vi "RANGE Configuration File.vi"(7 "Debug":bool, 8 "Error In":errorcluster, 11 "Gas Lab Config File":path=path "C:/Technology Lab/NI-2010/Trunk/Range/Documentation/GasLabConfigurationFile.txt") -> (0 "Error Out":errorcluster, 3 "Meter Data":T2={"Meter 1"={"Meter Size"=0.0, "DAQ Output (Voltage)"=0.0, "Reference (Voltage)"=0.0, "Meter Present"=FALSE, "Meter Visa"="COM3", "Gas Type"="", "SLPM Error @ Zero"=0.0, "Gas Mix Number"="", "Set STP Register"=FALSE, "Measurement Units"={"Abs. Pressure"="", "Gauge/Diff. Press."="", "Barometric Press."="", "Temperature"="", "Volume"="", "Mass"="", "Setpoint"="", "Valve Drive"="", "Totalizer"="", "Tot. Timer"="", "Tot. Avg. Flow"="", "Tot. Peak Flow"="", "Software Version"=""}}, "Meter 2"={"Meter Size"=0.0, "DAQ Output (Voltage)"=0.0, "Reference (Voltage)"=0.0, "Meter Present"=FALSE, "Meter Visa"="COM3", "Gas Type"="", "SLPM Error @ Zero"=0.0, "Gas Mix Number"="", "Set STP Register"=FALSE, "Measurement Units"={"Abs. Pressure"="", "Gauge/Diff. Press."="", "Barometric Press."="", "Temperature"="", "Volume"="", "Mass"="", "Setpoint"="", "Valve Drive"="", "Totalizer"="", "Tot. Timer"="", "Tot. Avg. Flow"="", "Tot. Peak Flow"="", "Software Version"=""}}, "Meter 3"={"Meter Size"=0.0, "DAQ Output (Voltage)"=0.0, "Reference (Voltage)"=0.0, "Meter Present"=FALSE, "Meter Visa"="COM3", "Gas Type"="", "SLPM Error @ Zero"=0.0, "Gas Mix Number"="", "Set STP Register"=FALSE, "Measurement Units"={"Abs. Pressure"="", "Gauge/Diff. Press."="", "Barometric Press."="", "Temperature"="", "Volume"="", "Mass"="", "Setpoint"="", "Valve Drive"="", "Totalizer"="", "Tot. Timer"="", "Tot. Avg. Flow"="", "Tot. Peak Flow"="", "Software Version"=""}}, "Meter 4"={"Meter Size"=0.0, "DAQ Output (Voltage)"=0.0, "Reference (Voltage)"=0.0, "Meter Present"=FALSE, "Meter Visa"="COM3", "Gas Type"="", "SLPM Error @ Zero"=0.0, "Gas Mix Number"="", "Set STP Register"=FALSE, "Measurement Units"={"Abs. Pressure"="", "Gauge/Diff. Press."="", "Barometric Press."="", "Temperature"="", "Volume"="", "Mass"="", "Setpoint"="", "Valve Drive"="", "Totalizer"="", "Tot. Timer"="", "Tot. Avg. Flow"="", "Tot. Peak Flow"="", "Software Version"=""}}, "Meter 5"={"Meter Size"=0.0, "DAQ Output (Voltage)"=0.0, "Reference (Voltage)"=0.0, "Meter Present"=FALSE, "Meter Visa"="COM3", "Gas Type"="", "SLPM Error @ Zero"=0.0, "Gas Mix Number"="", "Set STP Register"=FALSE, "Measurement Units"={"Abs. Pressure"="", "Gauge/Diff. Press."="", "Barometric Press."="", "Temperature"="", "Volume"="", "Mass"="", "Setpoint"="", "Valve Drive"="", "Totalizer"="", "Tot. Timer"="", "Tot. Avg. Flow"="", "Tot. Peak Flow"="", "Software Version"=""}}, "Meter 6"={"Meter Size"=0.0, "DAQ Output (Voltage)"=0.0, "Reference (Voltage)"=0.0, "Meter Present"=FALSE, "Meter Visa"="COM3", "Gas Type"="", "SLPM Error @ Zero"=0.0, "Gas Mix Number"="", "Set STP Register"=FALSE, "Measurement Units"={"Abs. Pressure"="", "Gauge/Diff. Press."="", "Barometric Press."="", "Temperature"="", "Volume"="", "Mass"="", "Setpoint"="", "Valve Drive"="", "Totalizer"="", "Tot. Timer"="", "Tot. Avg. Flow"="", "Tot. Peak Flow"="", "Software Version"=""}}, "Meter Bank 1"={"Flow Rate (BTU/HR)"=0.0, "ANSI Placeholder Array"=[], "15 Sec Avg Array"=[], "30 Sec Avg Array "=[], "ANSI Average (BTU/HR)"=0.0, "Panel Data"={"Meter Type (Gas)"="", "Heating Value (BTU/ft³)"=0.0, "Ft³ / Hr (SCFH)"=0.0, "15 Second Average (BTU/HR)"=0.0, "30 Second Average (BTU/HR)"=0.0, "Mass Flow"=0.0, "Vol. Flow"=0.0, "Gas Temperature"=0.0, "Gas Pressure"=0.0, "Tot.Flow"=0.0}, "Start ANSI"=FALSE, "ANSI Start Time"=0.0, "Restart ANSI"=FALSE, "Meter ID"=""}, "Meter Bank 2"={"Flow Rate (BTU/HR)"=0.0, "ANSI Placeholder Array"=[], "15 Sec Avg Array"=[], "30 Sec Avg Array "=[], "ANSI Average (BTU/HR)"=0.0, "Panel Data"={"Meter Type (Gas)"="", "Heating Value (BTU/ft³)"=0.0, "Ft³ / Hr (SCFH)"=0.0, "15 Second Average (BTU/HR)"=0.0, "30 Second Average (BTU/HR)"=0.0, "Mass Flow"=0.0, "Vol. Flow"=0.0, "Gas Temperature"=0.0, "Gas Pressure"=0.0, "Tot.Flow"=0.0}, "Start ANSI"=FALSE, "ANSI Start Time"=0.0, "Restart ANSI"=FALSE, "Meter ID"=""}, "Meter Bank 3"={"Flow Rate (BTU/HR)"=0.0, "ANSI Placeholder Array"=[], "15 Sec Avg Array"=[], "30 Sec Avg Array "=[], "ANSI Average (BTU/HR)"=0.0, "Panel Data"={"Meter Type (Gas)"="", "Heating Value (BTU/ft³)"=0.0, "Ft³ / Hr (SCFH)"=0.0, "15 Second Average (BTU/HR)"=0.0, "30 Second Average (BTU/HR)"=0.0, "Mass Flow"=0.0, "Vol. Flow"=0.0, "Gas Temperature"=0.0, "Gas Pressure"=0.0, "Tot.Flow"=0.0}, "Start ANSI"=FALSE, "ANSI Start Time"=0.0, "Restart ANSI"=FALSE, "Meter ID"=""}, "Threshold Voltage (NI DAQ)"=0.2, "Use RS232 Data Collection"=FALSE, "Use Auto Switching"=FALSE})   [LabVIEW 2018]
uses:
  Type Definitions/RANGE DAQ Data Four Meters.ctl
  Type Definitions/RANGE DAQ Data.ctl
  Drivers/Omega FMA-1600A Series Gas Flow Meter/Type Definitions/FMA1600A Gas Type.ctl
  Drivers/Omega FMA-1600A Series Gas Flow Meter/Type Definitions/FMA1600A Units String.ctl
  Type Definitions/RANGE GAS Data.ctl
  Type Definitions/RANGE Panel Data.ctl
panel:
  out "Meter 1.Measurement Units":T1
  out "all rows":string[][](array[string])
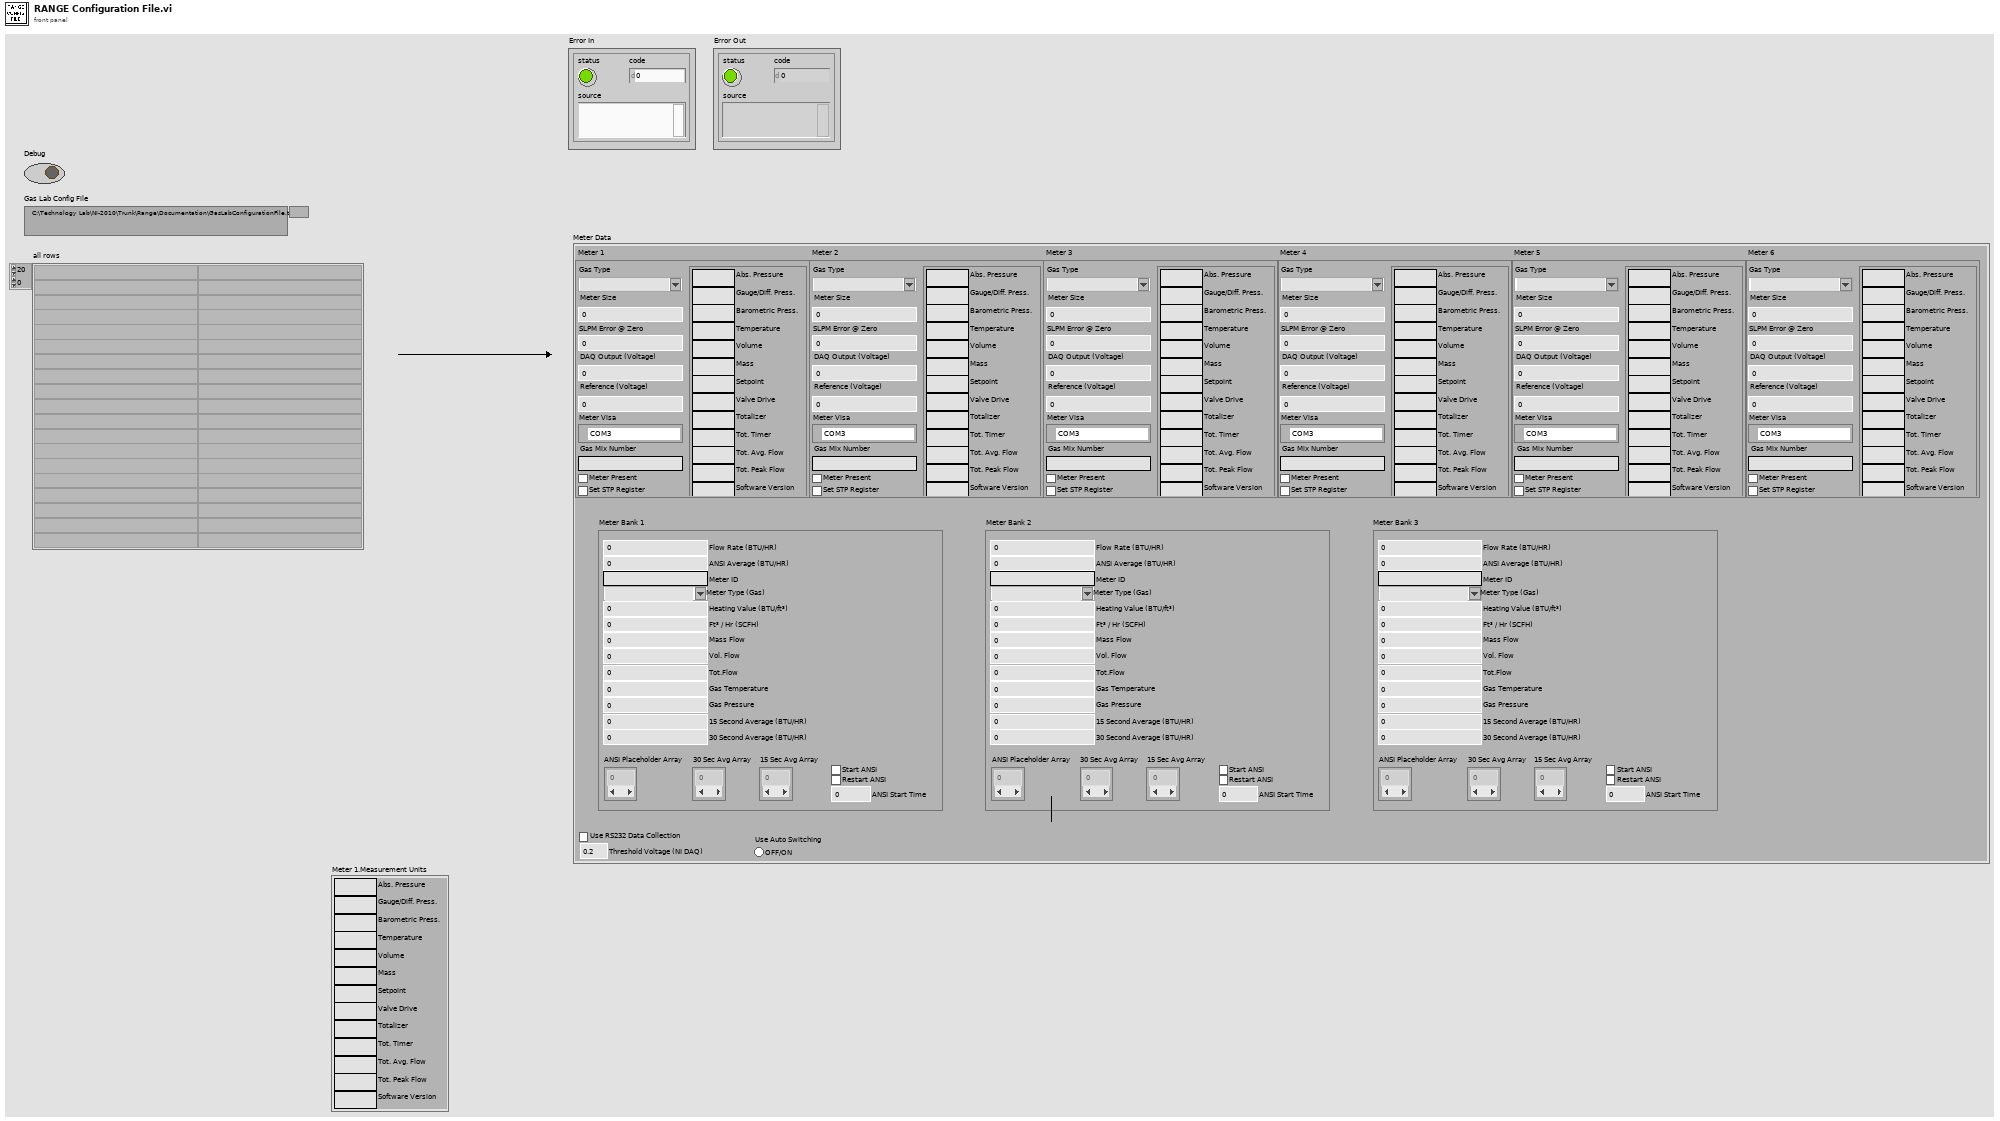
[diagram p1: front panel]
types:
  T1 = typedef "FMA1600A Units String.ctl" = cluster{"Abs. Pressure":string, "Gauge/Diff. Press.":string, "Barometric Press.":string, "Temperature":string, "Volume":string, "Mass":string, "Setpoint":string, "Valve Drive":string, "Totalizer":string, "Tot. Timer":string, "Tot. Avg. Flow":string, "Tot. Peak Flow":string, "Software Version":string}
  T2 = typedef "RANGE DAQ Data Four Meters.ctl" = cluster{"Meter 1":T3, "Meter 2":T3, "Meter 3":T3, "Meter 4":T3, "Meter 5":T3, "Meter 6":T3, "Meter Bank 1":T5, "Meter Bank 2":T5, "Meter Bank 3":T5, "Threshold Voltage (NI DAQ)":dbl, "Use RS232 Data Collection":bool, "Use Auto Switching":bool}
  T3 = typedef "RANGE DAQ Data.ctl" = cluster{"Meter Size":dbl, "DAQ Output (Voltage)":dbl, "Reference (Voltage)":dbl, "Meter Present":bool, "Meter Visa":refnum<visa-resource-name>, "Gas Type":T4, "SLPM Error @ Zero":dbl, "Gas Mix Number":string, "Set STP Register":bool, "Measurement Units":T1}
  T4 = typedef "FMA1600A Gas Type.ctl" = string
  T5 = typedef "RANGE GAS Data.ctl" = cluster{"Flow Rate (BTU/HR)":dbl, "ANSI Placeholder Array":dbl[], "15 Sec Avg Array":dbl[], "30 Sec Avg Array ":dbl[], "ANSI Average (BTU/HR)":dbl, "Panel Data":T6, "Start ANSI":bool, "ANSI Start Time":dbl, "Restart ANSI":bool, "Meter ID":string}
  T6 = typedef "RANGE Panel Data.ctl" = cluster{"Meter Type (Gas)":T4, "Heating Value (BTU/ft³)":dbl, "Ft³ / Hr (SCFH)":dbl, "15 Second Average (BTU/HR)":dbl, "30 Second Average (BTU/HR)":dbl, "Mass Flow":dbl, "Vol. Flow":dbl, "Gas Temperature":dbl, "Gas Pressure":dbl, "Tot.Flow":dbl}
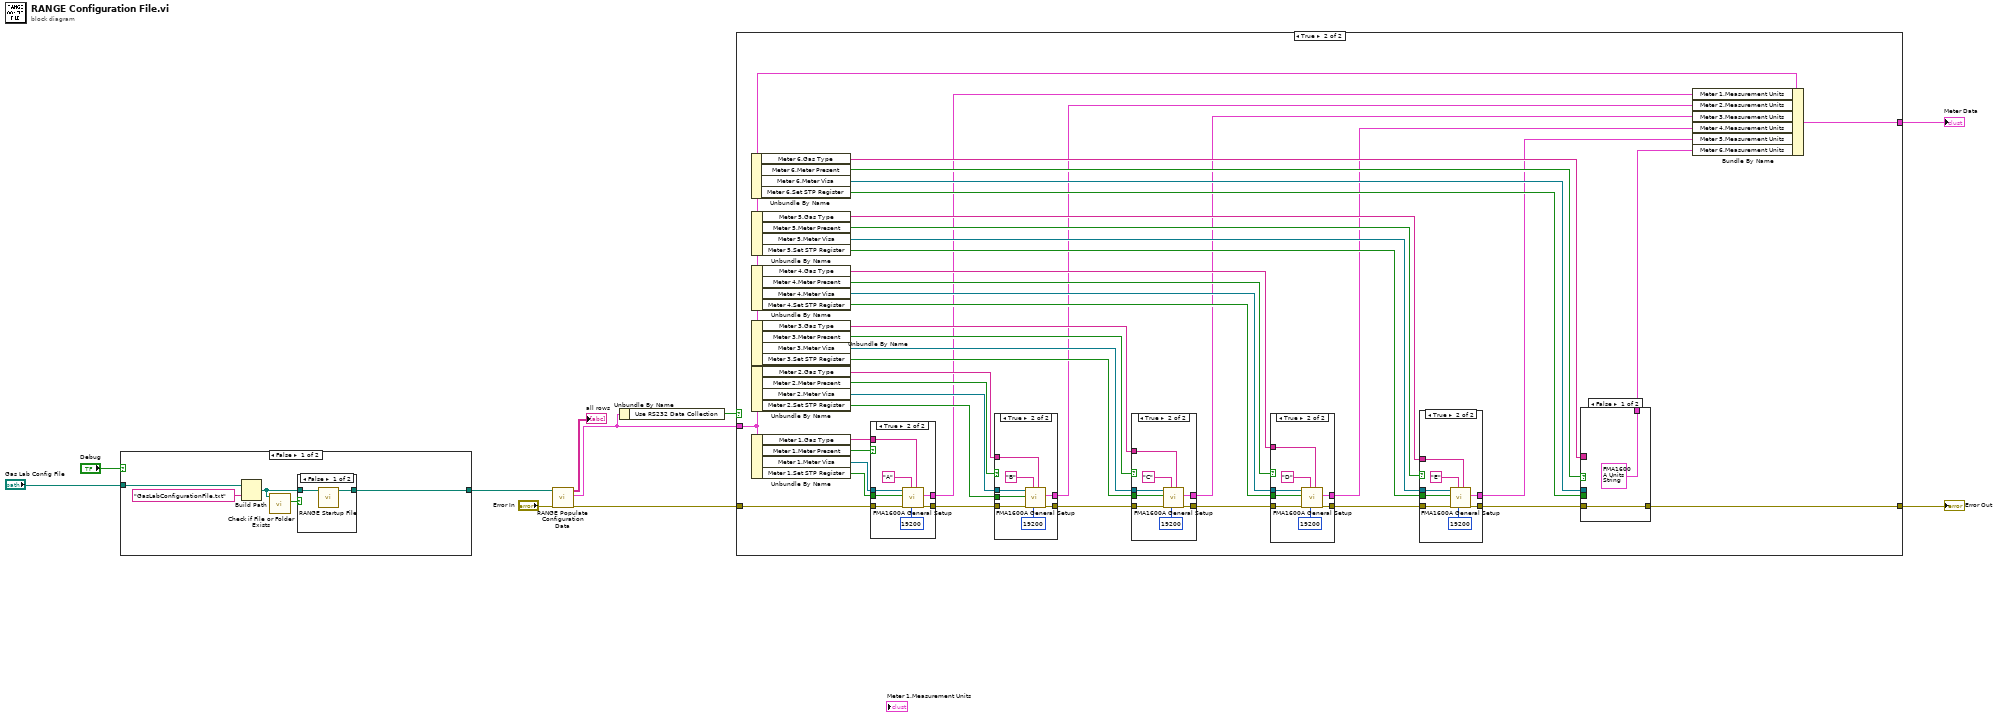
[diagram p0: block diagram]
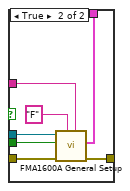
[diagram p3: hidden frame]
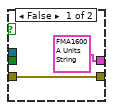
[diagram p4: hidden frame]
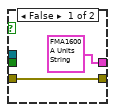
[diagram p5: hidden frame]
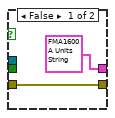
[diagram p6: hidden frame]
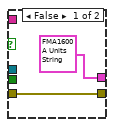
[diagram p7: hidden frame]
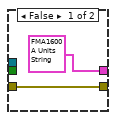
[diagram p8: hidden frame]
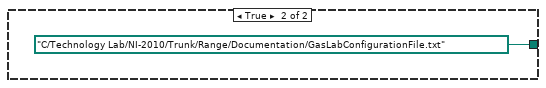
[diagram p10: hidden frame]
diagram:
  n1 = case shown="False" "Debug" {
    tunnel: "Gas Lab Config File" -> [w15 _]
    tunnel: [w11 path "C:/Technology Lab/NI-2010/Trunk/Range/Documentation/GasLabConfigurationFile.txt" ("appended path")] -> w8
    frame False {
      n2 = Build Path(base path=w15, name or relative path="GasLabConfigurationFile.txt") -> (appended path=w12:path)
      n3 = call <vilib>:"Check if File or Folder Exists.vi"("path"=w12) -> ("file or folder exists?"=w13:bool)  [unwired: 8 in, 2 out]
      n4 = case shown="False" w13 {
        tunnel: w12 -> [w17 w18]
        tunnel: [w16 w18] -> w11
        frame False {
          n5 = call "RANGE Startup File.vi"("appended path"=w17) -> ("new file path (Not A Path if cancelled)"=w16:path)  [unwired: 10 in]
        }
        frame True {
        }
      }
    }
    frame True {
    }
  }
  n6 = call "RANGE Populate Configuration Data.vi"("error in (no error)"="Error In", "appended path"=w8) -> ("error out"=w5:errorcluster, "DAQ Data"=w3:T2, "all rows"=→"all rows":string[][])  [unwired: 7 in]
  n7 = Unbundle By Name(w3) -> ("Use RS232 Data Collection"=w4:bool)
  n8 = case shown="True" w4 {
    tunnel: w5 -> [w21 w60]
    tunnel: w3 -> [w20 w29]
    tunnel: [w21 w52] -> w2
    tunnel: [w20 w22] -> w1
    frame False {
    }
    frame True {
      n9 = Unbundle By Name(w29) -> ("Meter 6.Gas Type"=w36:T4, "Meter 6.Meter Present"=w43:bool, "Meter 6.Meter Visa"=w42:refnum<visa-resource-name>, "Meter 6.Set STP Register"=w30:bool)
      n10 = Unbundle By Name(w29) -> ("Meter 5.Gas Type"=w37:T4, "Meter 5.Meter Present"=w45:bool, "Meter 5.Meter Visa"=w44:refnum<visa-resource-name>, "Meter 5.Set STP Register"=w31:bool)
      n11 = Unbundle By Name(w29) -> ("Meter 4.Gas Type"=w38:T4, "Meter 4.Meter Present"=w47:bool, "Meter 4.Meter Visa"=w46:refnum<visa-resource-name>, "Meter 4.Set STP Register"=w32:bool)
      n12 = Unbundle By Name(w29) -> ("Meter 3.Gas Type"=w39:T4, "Meter 3.Meter Present"=w49:bool, "Meter 3.Meter Visa"=w48:refnum<visa-resource-name>, "Meter 3.Set STP Register"=w33:bool)
      n13 = Unbundle By Name(w29) -> ("Meter 2.Gas Type"=w40:T4, "Meter 2.Meter Present"=w51:bool, "Meter 2.Meter Visa"=w50:refnum<visa-resource-name>, "Meter 2.Set STP Register"=w34:bool)
      n14 = Unbundle By Name(w29) -> ("Meter 1.Gas Type"=w41:T4, "Meter 1.Meter Present"=w59:bool, "Meter 1.Meter Visa"=w58:refnum<visa-resource-name>, "Meter 1.Set STP Register"=w35:bool)
      n15 = case shown="True" w59 {
        tunnel: w60 -> [w111 w119]
        tunnel: w58 -> [_ w118]
        tunnel: [w111 w116] -> w57
        tunnel: w41 -> [_ w115]
        tunnel: w35 -> [_ w114]
        tunnel: [T1 {"Abs. Pressure"="", "Gauge/Diff. Press."="", "Barometric Press."="", "Temperature"="", "Volume"="", "Mass"="", "Setpoint"="", "Valve Drive"="", "Totalizer"="", "Tot. Timer"="", "Tot. Avg. Flow"="", "Tot. Peak Flow"="", "Software Version"=""} ("Measurement Units") w113] -> w28
        frame False {
        }
        frame True {
          n16 = call "FMA1600A General Setup.vi"("Gas Type"=w115, "baud rate (19200)"=u32 19200, "Unit ID"="A", "error in (no error)"=w119, "Set STP Register"=w114, "VISA Refnum in"=w118) -> ("error out"=w116:errorcluster, "Measurement Units"=w113:T1)  [unwired: 3 in, 1 out]
        }
      }
      n17 = case shown="True" w51 {
        tunnel: w57 -> [w101 w109]
        tunnel: w50 -> [_ w108]
        tunnel: [w101 w106] -> w56
        tunnel: w40 -> [_ w105]
        tunnel: w34 -> [_ w104]
        tunnel: [T1 {"Abs. Pressure"="", "Gauge/Diff. Press."="", "Barometric Press."="", "Temperature"="", "Volume"="", "Mass"="", "Setpoint"="", "Valve Drive"="", "Totalizer"="", "Tot. Timer"="", "Tot. Avg. Flow"="", "Tot. Peak Flow"="", "Software Version"=""} ("Measurement Units") w103] -> w27
        frame False {
        }
        frame True {
          n18 = call "FMA1600A General Setup.vi"("Gas Type"=w105, "baud rate (19200)"=u32 19200, "Unit ID"="B", "error in (no error)"=w109, "Set STP Register"=w104, "VISA Refnum in"=w108) -> ("error out"=w106:errorcluster, "Measurement Units"=w103:T1)  [unwired: 3 in, 1 out]
        }
      }
      n19 = case shown="True" w49 {
        tunnel: w56 -> [w91 w99]
        tunnel: w48 -> [_ w98]
        tunnel: [w91 w96] -> w55
        tunnel: w39 -> [_ w95]
        tunnel: w33 -> [_ w94]
        tunnel: [T1 {"Abs. Pressure"="", "Gauge/Diff. Press."="", "Barometric Press."="", "Temperature"="", "Volume"="", "Mass"="", "Setpoint"="", "Valve Drive"="", "Totalizer"="", "Tot. Timer"="", "Tot. Avg. Flow"="", "Tot. Peak Flow"="", "Software Version"=""} ("Measurement Units") w93] -> w26
        frame False {
        }
        frame True {
          n20 = call "FMA1600A General Setup.vi"("Gas Type"=w95, "baud rate (19200)"=u32 19200, "Unit ID"="C", "error in (no error)"=w99, "Set STP Register"=w94, "VISA Refnum in"=w98) -> ("error out"=w96:errorcluster, "Measurement Units"=w93:T1)  [unwired: 3 in, 1 out]
        }
      }
      n21 = case shown="True" w47 {
        tunnel: w55 -> [w81 w89]
        tunnel: w46 -> [_ w88]
        tunnel: [w81 w86] -> w54
        tunnel: w38 -> [_ w85]
        tunnel: w32 -> [_ w84]
        tunnel: [T1 {"Abs. Pressure"="", "Gauge/Diff. Press."="", "Barometric Press."="", "Temperature"="", "Volume"="", "Mass"="", "Setpoint"="", "Valve Drive"="", "Totalizer"="", "Tot. Timer"="", "Tot. Avg. Flow"="", "Tot. Peak Flow"="", "Software Version"=""} ("Measurement Units") w83] -> w25
        frame False {
        }
        frame True {
          n22 = call "FMA1600A General Setup.vi"("Gas Type"=w85, "baud rate (19200)"=u32 19200, "Unit ID"="D", "error in (no error)"=w89, "Set STP Register"=w84, "VISA Refnum in"=w88) -> ("error out"=w86:errorcluster, "Measurement Units"=w83:T1)  [unwired: 3 in, 1 out]
        }
      }
      n23 = case shown="True" w45 {
        tunnel: w54 -> [w71 w79]
        tunnel: w44 -> [_ w78]
        tunnel: [w71 w76] -> w53
        tunnel: w37 -> [_ w75]
        tunnel: w31 -> [_ w74]
        tunnel: [T1 {"Abs. Pressure"="", "Gauge/Diff. Press."="", "Barometric Press."="", "Temperature"="", "Volume"="", "Mass"="", "Setpoint"="", "Valve Drive"="", "Totalizer"="", "Tot. Timer"="", "Tot. Avg. Flow"="", "Tot. Peak Flow"="", "Software Version"=""} ("Measurement Units") w73] -> w24
        frame False {
        }
        frame True {
          n24 = call "FMA1600A General Setup.vi"("Gas Type"=w75, "baud rate (19200)"=u32 19200, "Unit ID"="E", "error in (no error)"=w79, "Set STP Register"=w74, "VISA Refnum in"=w78) -> ("error out"=w76:errorcluster, "Measurement Units"=w73:T1)  [unwired: 3 in, 1 out]
        }
      }
      n25 = case shown="False" w43 {
        tunnel: w53 -> [w62 w69]
        tunnel: w42 -> [_ w68]
        tunnel: [w62 w66] -> w52
        tunnel: w36 -> [_ w65]
        tunnel: w30 -> [_ w64]
        tunnel: [T1 {"Abs. Pressure"="", "Gauge/Diff. Press."="", "Barometric Press."="", "Temperature"="", "Volume"="", "Mass"="", "Setpoint"="", "Valve Drive"="", "Totalizer"="", "Tot. Timer"="", "Tot. Avg. Flow"="", "Tot. Peak Flow"="", "Software Version"=""} ("Measurement Units") w63] -> w23
        frame False {
        }
        frame True {
          n26 = call "FMA1600A General Setup.vi"("Gas Type"=w65, "Unit ID"="F", "error in (no error)"=w69, "Set STP Register"=w64, "VISA Refnum in"=w68) -> ("error out"=w66:errorcluster, "Measurement Units"=w63:T1)  [unwired: 4 in, 1 out]
        }
      }
      n27 = Bundle By Name(cluster=w29, "Meter 1.Measurement Units"=w28, "Meter 2.Measurement Units"=w27, "Meter 3.Measurement Units"=w26, "Meter 4.Measurement Units"=w25, "Meter 5.Measurement Units"=w24, "Meter 6.Measurement Units"=w23) -> (w22:T2)
    }
  }
  "Meter Data" <- w1
  "Error Out" <- w2
